vi "SLL DE AI LV2 Global.vi"(6 "AI value Array":dbl[](array[numeric]), 7 "AI Option":T2, 8 "error in (no error)":errorcluster, 9 "AI value":dbl, 10 "AI Channel Name Array":T1[](array[typedef]), 11 "AI Channel Name":T1) -> (0 "error out":errorcluster, 2 "Analog Input Array Value":dbl[](array[numeric]), 3 "Analog Input Line Value":dbl)   [LabVIEW 2013]
uses:
  Controls/SLL DE AI Global Options.ctl
  Controls/SLL DE List of Analog Inputs.ctl
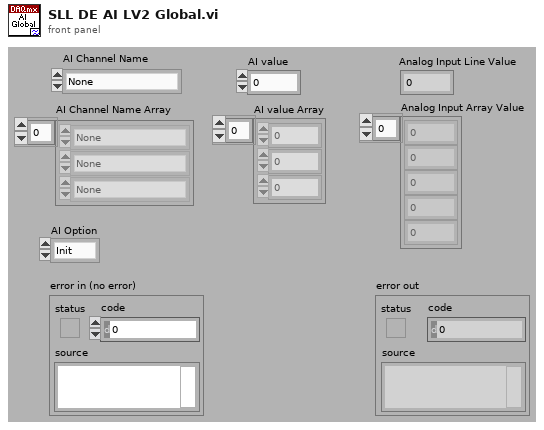
[diagram p1: front panel]
types:
  T1 = typedef "SLL DE List of Analog Inputs.ctl" = enum16{"None"}
  T2 = typedef "SLL DE AI Global Options.ctl" = enum16{"Init", "Write Line", "Write Array", "Read Line", "Read Array", "Read Full Status", "Write Full Status"}
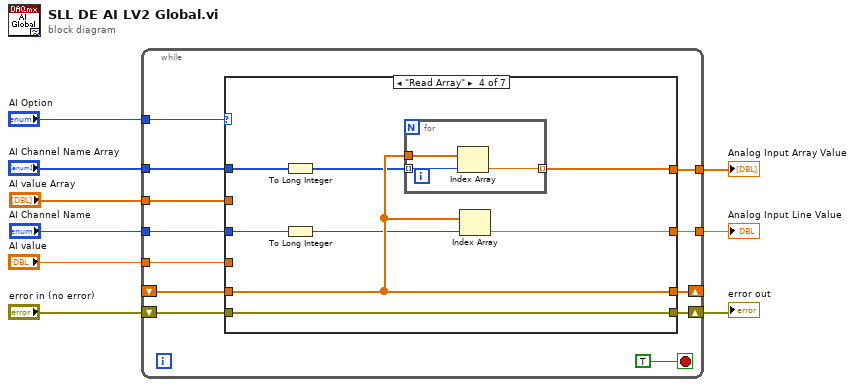
[diagram p0: block diagram]
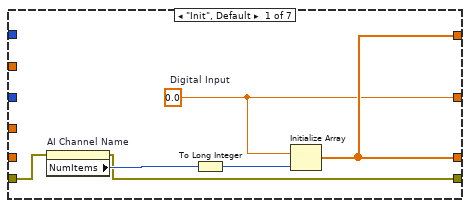
[diagram p2: hidden frame]
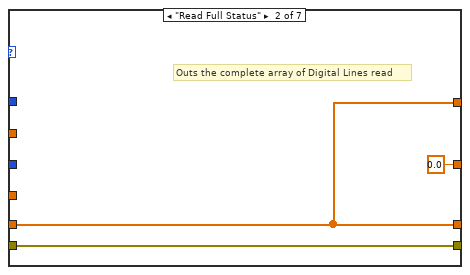
[diagram p3: hidden frame]
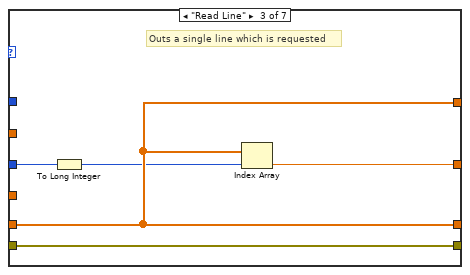
[diagram p4: hidden frame]
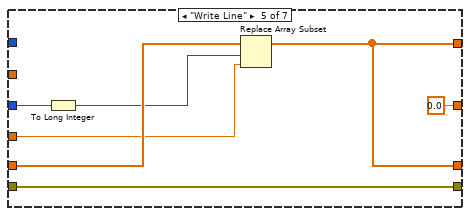
[diagram p5: hidden frame]
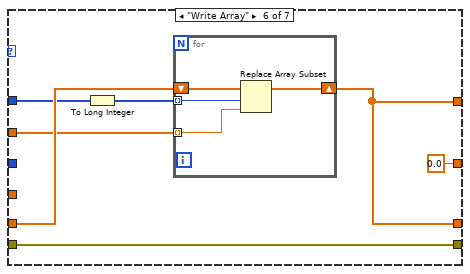
[diagram p6: hidden frame]
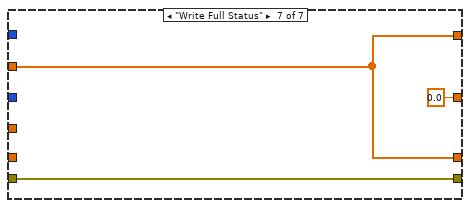
[diagram p7: hidden frame]
diagram:
  n1 = while {
    shift-right: [w20] -> _
    shift-left: _ -> [w19]
    tunnel: "AI Channel Name Array" -> [w18]
    tunnel: "AI Channel Name" -> [w17]
    tunnel: [w16] -> w7
    tunnel: [w15] -> w6
    shift-right: [w13] -> w4
    shift-left: "error in (no error)" -> [w14]
    tunnel: "AI value Array" -> [w12]
    tunnel: "AI value" -> [w11]
    tunnel: "AI Option" -> [w10]
    stop <- TRUE stop-if-true
    n2 = case shown="\"Read Array\"" w10 {
      tunnel: [w27 w30 w33 w40 w53 w60 w65] -> w20
      tunnel: w19 -> [_ w30 w33 w40 w51 w58 _]
      tunnel: w18 -> [_ _ _ w43 _ w56 _]
      tunnel: w17 -> [_ _ w35 w39 w49 _ _]
      tunnel: [w26 0.0 ("Digital Input") w34 w38 0.0 ("Digital Input") 0.0 ("Digital Input") 0.0 ("Digital Input")] -> w16
      tunnel: [w27 w30 w33 w42 w53 w60 w65] -> w15
      tunnel: w14 -> [w24 w29 w32 w41 w52 w59 w67]
      tunnel: [w23 w29 w32 w41 w52 w59 w67] -> w13
      tunnel: w12 -> [_ _ _ _ _ w57 w65]
      tunnel: w11 -> [_ _ _ _ w50 _ _]
      frame "Init", Default {
        w26 = 0.0  # Digital Input
        n3 = property on="AI Channel Name" class="Enum (strict)"(error in=w24) -> (error out=w23:errorcluster, "NumItems"=w25:u32)  [unwired: 1 in, 1 out]
        n4 = To Long Integer(number=w25) -> (32bit integer=w22:i32)
        n5 = Initialize Array(w26, w22) -> (w27:dbl[])
      }
      frame "Read Full Status" {
        # "Outs the complete array of Digital Lines read"
      }
      frame "Read Line" {
        # "Outs a single line which is requested"
        n6 = To Long Integer(number=w35) -> (32bit integer=w31:i32)
        n7 = Index Array(array=w33, index=w31) -> (element=w34:dbl)
      }
      frame "Read Array" {
        n8 = To Long Integer(number=w43) -> (32bit integer=w36:i32[])
        n9 = To Long Integer(number=w39) -> (32bit integer=w37:i32)
        n10 = for {
          tunnel: w40 -> [w46]
          tunnel: w36 -> [w45] mode=indexing
          tunnel: [w44] -> w42 mode=indexing
          n11 = Index Array(array=w46, index=w45) -> (element=w44:dbl)
        }
        n12 = Index Array(array=w40, index=w37) -> (element=w38:dbl)
      }
      frame "Write Line" {
        n13 = To Long Integer(number=w49) -> (32bit integer=w48:i32)
        n14 = Replace Array Subset(array=w51, new element=w50, index=w48) -> (w53:dbl[])
      }
      frame "Write Array" {
        n15 = To Long Integer(number=w56) -> (32bit integer=w55:i32[])
        n16 = for {
          tunnel: w57 -> [w62] mode=indexing
          shift-right: [w63] -> w60
          shift-left: w58 -> [w64]
          tunnel: w55 -> [w61] mode=indexing
          n17 = Replace Array Subset(array=w64, new element=w62, index=w61) -> (w63:dbl[])
        }
      }
      frame "Write Full Status" {
      }
    }
  }
  "error out" <- w4
  "Analog Input Line Value" <- w7
  "Analog Input Array Value" <- w6
